vi "NXT_HINDBRAIN Build Message String.vi"(1 "_sensorData":T2={"_irData"={"_irDistance"=0, "_irHeading"=0, "_irTimestamp"=0}, "_batteryVoltage"=0, "_NXTButtonStates"=[FALSE, FALSE, FALSE]}, 2 "_motorCommands":T1={"_rudderCommand"=7, "_propCommand"=7, "_irServoCommand"=7}) -> (0 "Data Out":string)   [LabVIEW 2012]
uses:
  sensorData_t.ctl
  irData_t.ctl
  motorCommands_t.ctl
panel:
  # "L\nE\nF\nT"
  # "C\nE\nN\nT\nE\nR"
  # "R\nI\nG\nH\nT"
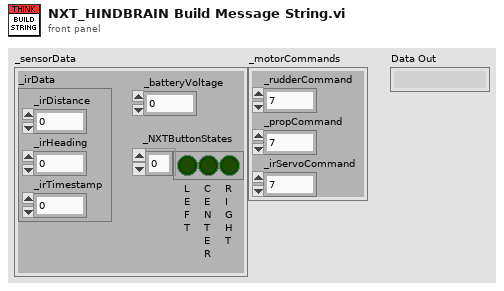
[diagram p1: front panel]
types:
  T1 = typedef "motorCommands_t.ctl" = cluster{"_rudderCommand":i8, "_propCommand":i8, "_irServoCommand":i8}
  T2 = typedef "sensorData_t.ctl" = cluster{"_irData":T3, "_batteryVoltage":i32, "_NXTButtonStates":bool[]}
  T3 = typedef "irData_t.ctl" = cluster{"_irDistance":i32, "_irHeading":i32, "_irTimestamp":u32}
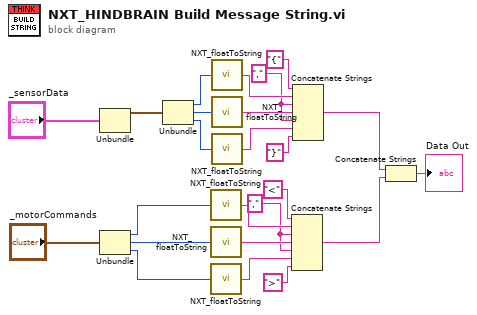
[diagram p0: block diagram]
diagram:
  w8 = "," ("string")
  w14 = "," ("string")
  n1 = Unbundle("_sensorData") -> ("_irData"=w22:T3)  [unwired: 2 out]
  n2 = Unbundle("_motorCommands") -> ("_rudderCommand"=w5:i8, "_propCommand"=w6:i8, "_irServoCommand"=w4:i8)
  n3 = Unbundle(w22) -> ("_irDistance"=w21:i32, "_irHeading"=w20:i32, "_irTimestamp"=w19:u32)
  n4 = call <vilib>:"NXT_floatToString.vi"("number"=w5) -> ("string"=w11:string)
  n5 = call <vilib>:"NXT_floatToString.vi"("number"=w6) -> ("string"=w10:string)
  n6 = call <vilib>:"NXT_floatToString.vi"("number"=w4) -> ("string"=w9:string)
  n7 = call <vilib>:"NXT_floatToString.vi"("number"=w21) -> ("string"=w17:string)
  n8 = call <vilib>:"NXT_floatToString.vi"("number"=w20) -> ("string"=w16:string)
  n9 = call <vilib>:"NXT_floatToString.vi"("number"=w19) -> ("string"=w15:string)
  n10 = Concatenate Strings("<" ("string"), w11, w8, w10, w8, w9, ">" ("string")) -> (w2:string)
  n11 = Concatenate Strings("{" ("string"), w17, w14, w16, w14, w15, "}" ("string")) -> (w3:string)
  n12 = Concatenate Strings(w3, w2) -> (→"Data Out":string)
